vi "Read U16 Array.vi"(10 "Size":u32, 11 "unsigned byte array":u8[](array[numeric])) -> (3 "U16 Array Out":u16[](array[numeric]), 5 "rest of array":u8[](array[numeric]))   [LabVIEW 2015]
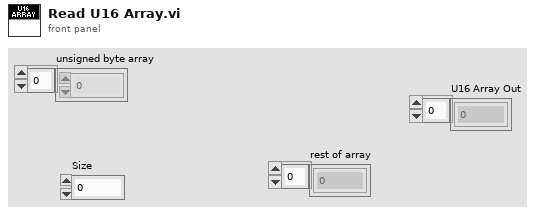
[diagram p1: front panel]
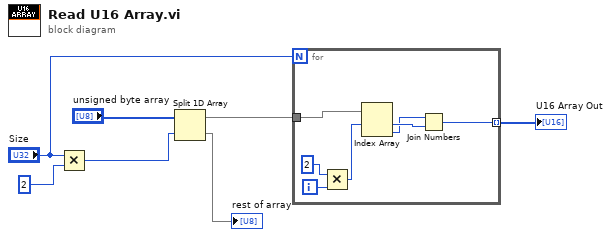
[diagram p0: block diagram]
diagram:
  n1 = Multiply(x="Size", y=u32 2) -> (x*y=w4:u32)
  n2 = Split 1D Array(array="unsigned byte array", index=w4) -> (first subarray=w2:u8[], second subarray=→"rest of array":u8[])
  n3 = for {
    N: "Size" -> [_]
    tunnel: w2 -> [w14]
    tunnel: [w8] -> w1 mode=indexing
    i -> [w13]
    n4 = Multiply(x=2, y=w13) -> (x*y=w11:i32)
    n5 = Index Array(array=w14, index #1=w11) -> (element #1=w10:u8, element #2=w9:u8)  [unwired: 1 in]
    n6 = Join Numbers(hi=w9, lo=w10) -> ((hi.lo)=w8:u16)
  }
  "U16 Array Out" <- w1
